vi "DSB Modulation Demo.vi"() -> ()   [LabVIEW 2013]
uses:
  <vilib>/express/express analysis/Spectral/Block/exnSpectralBlock spectral measurements RMS poly.vi
  <vilib>/express/express analysis/Spectral/Block/exnSpectralBlock spectral measurements RMS DDT.vi
  <vilib>/express/express analysis/Spectral/XNode/ExpressSpectralMeasurementsBlockNode.xnode
panel:
  out "Estimated Freq.":dbl caption="Amplitude" format="%#_9g"
  in  "WAV Sample Rate":dbl=44100.0 caption="dt"
  in  "Modulation Freq.":dbl=2000.0 caption="Frequency"
  in  "LPF Cut-Off":dbl=10000.0 caption="Lower Cut-Off"
  in  "SNR (dB)":dbl(slide)=30.0 caption="Standard deviation" scale=-20.0..30.0
  out "Comparision":dynamicdata(graph)
  out "Baseband":dynamicdata(graph)
  out "DSB FFT":dynamicdata(graph)
  out "DSB Wave":dynamicdata(graph)
  in  "Carrier Amp.":dbl=1.0 caption="Amplitude"
  in  "stop":bool
  in  "Frequency Offset":dbl(slide) scale=0.0..1000.0
  in  "Carrier Freq.":dbl=100000.0 caption="Frequency"
  # "DSB Modulation"
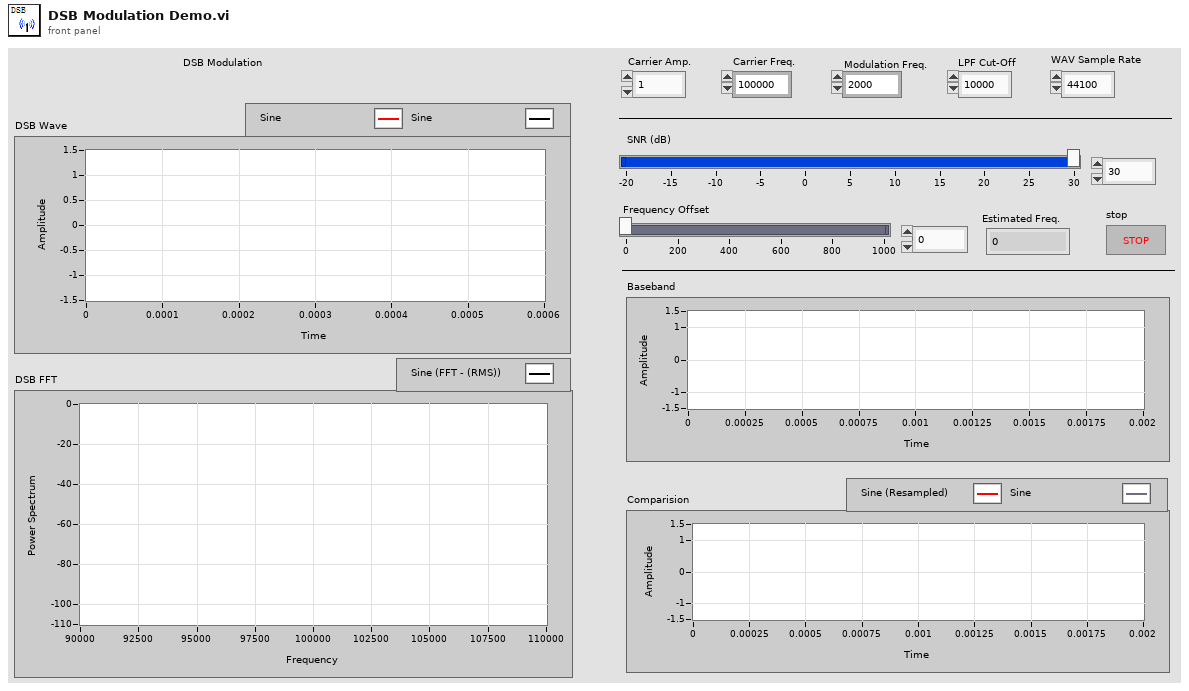
[diagram p1: front panel]
types:
  T1 = cluster{"averaging mode":u16, "weighting mode":u16, "number of averages":u32}
  T2 = cluster{"dB On (F)":bool, "unwrap phase (F)":bool, "convert to degree (F)":bool}
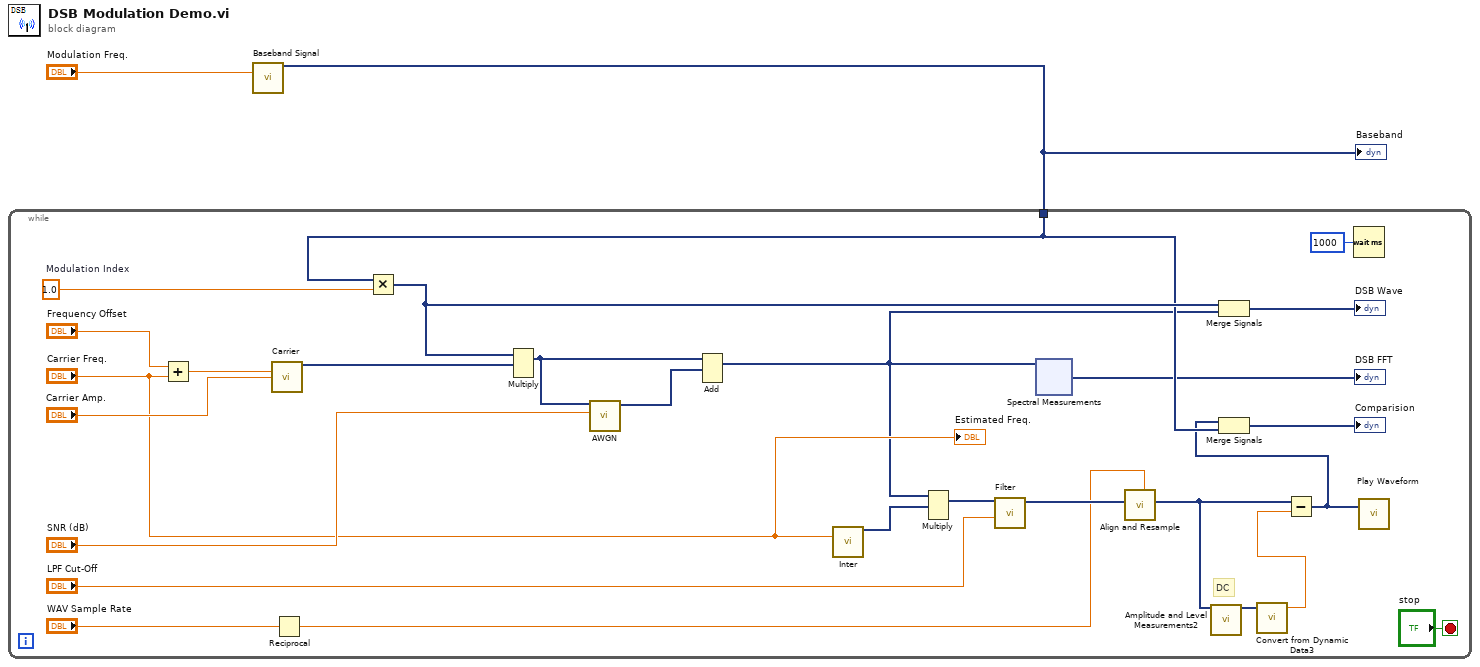
[diagram p0: block diagram]
diagram:
  n1 = call "Baseband Signal"("Frequency"="Modulation Freq.") -> ("Sine"=w1:dynamicdata)  [unwired: 13 in, 1 out]
  "Baseband" <- w1
  n2 = while {
    tunnel: w1 -> [w10]
    stop <- "stop" stop-if-true
    w23 = 1.0  # Modulation Index
    # "DC"
    n3 = Add(x="Frequency Offset", y="Carrier Freq.") -> (x+y=w22:dbl)
    n4 = call "Carrier"("Frequency"=w22, "Amplitude"="Carrier Amp.") -> ("Sine"=w19:dynamicdata)  [unwired: 12 in, 1 out]
    n5 = Reciprocal(x="WAV Sample Rate") -> (1/x=w12:dbl)
    n6 = Multiply(x=w10, y=w23) -> (x*y=w18:dynamicdata)
    n7 = Multiply(1:w19, 2:w18) -> (0:w17:dynamicdata)  [unwired: 1 in, 1 out]
    n8 = call "AWGN.vi"("SNR (dB)"="SNR (dB)", "Dynamic Data"=w17) -> ("DC with Gaussian Noise"=w16:dynamicdata)  [unwired: 9 in]
    n9 = Add(1:w16, 2:w17) -> (0:w3:dynamicdata)  [unwired: 1 in, 1 out]
    n10 = call "Inter"("Frequency"="Carrier Freq.") -> ("Sine"=w4:dynamicdata)  [unwired: 13 in, 1 out]
    n11 = Multiply(1:w4, 2:w3) -> (0:w6:dynamicdata)  [unwired: 1 in, 1 out]
    n12 = call "Filter"("Lower Cut-Off"="LPF Cut-Off", "Signal"=w6) -> ("Filtered Signal"=w14:dynamicdata)  [unwired: 8 in, 1 out]
    n13 = xnode ("Spectral Measurements")("Signals"=w3) -> ("FFT - (RMS)"=→"DSB FFT":dynamicdata)  [unwired: 1 in, 2 out]
    n14 = call "Align and Resample"("dt"=w12, "Signals"=w14) -> ("Resampled Signals"=w26:dynamicdata)  [unwired: 7 in, 2 out]
    n15 = call "Amplitude and Level Measurements2"("Signals"=w26) -> ("Mean (DC)"=w28:dynamicdata)  [unwired: 13 in, 1 out]
    n16 = Merge Signals(w18, w3) -> (→"DSB Wave":dynamicdata)
    n17 = call "Convert from Dynamic Data3"("Dynamic Data Type"=w28) -> ("Scalar"=w25:dbl)  [unwired: 3 in]
    n18 = Subtract(x=w26, y=w25) -> (x-y=w9:dynamicdata)
    n19 = Merge Signals(w9, w10) -> (→"Comparision":dynamicdata)
    n20 = Wait (ms)(milliseconds to wait=u32 1000) -> ()  [unwired: 1 out]
    n21 = call "Play Waveform"("Data"=w9) -> ()  [unwired: 18 in, 1 out]
    "Estimated Freq." <- "Carrier Freq."
  }
